vi "Configure Dispense Mode.vi"(8 "error in (no error)":errorcluster, 10 "Dispense Mode (0: Steady)":u16(ring) items=["Steady Mode", "Timed Mode"], 11 "VISA resource name":refnum<visa-resource-name>) -> (0 "error out":errorcluster, 3 "VISA resource name out":refnum<visa-resource-name>)   [LabVIEW 2018, in "EFD Ultimus V.lvlib"]
doc: "This VI switches the dispenser into Timed Mode or Steady Mode.\nTimed Mode:\n Host Format: TT--\nSteady Mode:\n Host Format: MT--"
uses:
  EFD Ultimus V.lvlib
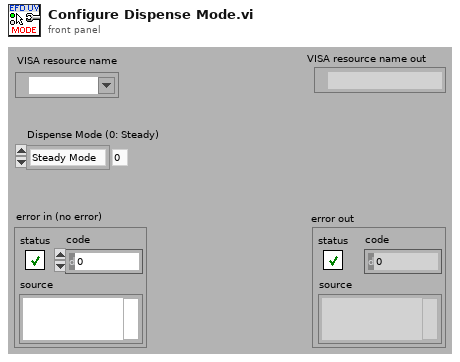
[diagram p1: front panel]
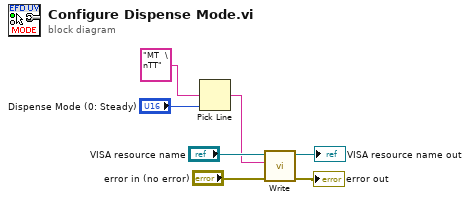
[diagram p0: block diagram]
diagram:
  n1 = Pick Line(multi-line string="MT  \nTT", line index="Dispense Mode (0: Steady)") -> (output string=w1:string)  [unwired: 1 in]
  n2 = call "Write.vi"("error in (no error)"="error in (no error)", "Command To Write"=w1, "VISA resource name"="VISA resource name") -> ("error out"=→"error out":errorcluster, "VISA resource name out"=→"VISA resource name out":refnum<visa-resource-name>)  [unwired: 7 out]
